vi "Init Resources.vi"(8 "Error In":errorcluster, 11 "WebView in":refnum<class "WebView.lvclass">) -> (0 "Error Out":errorcluster, 3 "WebView out":refnum<class "WebView.lvclass">)   [LabVIEW 2024, in "WebView.lvclass"]
uses:
  WebView.lvclass/WebView.ctl
  WebView.lvclass
  <vilib>/sklein/WebView2/Libs/Microsoft.Web.WebView2.Core.dll
  Resources--cluster.ctl
  <vilib>/sklein/WebView2/Libs/Microsoft.Web.WebView2.WinForms.dll
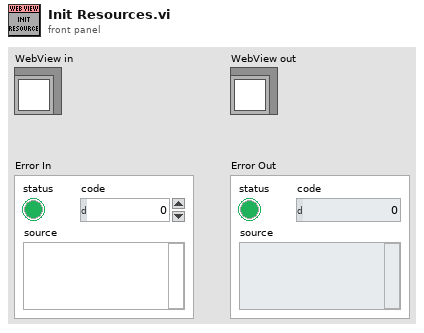
[diagram p1: front panel]
types:
  T1 = typedef "WebView.lvclass/Resources--cluster.ctl" = cluster{"WebView2 Control":refnum<k24>, "Webview2 Core":refnum<k24>, "event callback":refnum<k27>, "Environment":refnum<k24>}
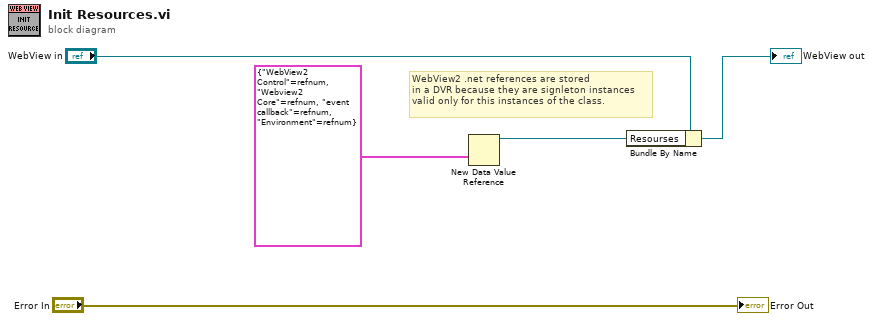
[diagram p0: block diagram]
diagram:
  # "WebView2 .net references are stored \nin a DVR because they are signleton instances\nvalid only for this instances of the class."
  n1 = New Data Value Reference(data value=T1 {"WebView2 Control"=refnum, "Webview2 Core"=refnum, "event callback"=refnum, "Environment"=refnum}) -> (data value reference=w4:refnum<data-value>)  [unwired: 1 in, 1 out]
  n2 = Bundle By Name(cluster="WebView in", "Resourses"=w4) -> (→"WebView out":refnum<class "WebView.lvclass">)
  "Error Out" <- "Error In"
